vi "ROS2.vi"(7 "JPG":refnum<vi>, 10 "queueName":string="PV_script", 11 "Console Reference":refnum<vi>) -> ()   [LabVIEW 2022 SP3]
uses:
  ROS_Subs/ROSCtrl.ctl
  <vilib>/Platform/browser.llb/Open URL in Default Browser (string).vi
panel:
  in  "Tab Control":T1(tab)
  in  "Cmds":T2
  in  "LightShow":u32[](array[colorbox])=[16711680, 327424, 393471, 15699456, 14811391, 64255]
  in  "LED Colors":u32[](array[colorbox])=[16711680, 327424, 393471, 15699456, 14811391, 64255]
  in  "LED Info":T3={"Node Name"="Node", "Topic Name"="/cmd_lightring", "Message Type"="irobot_create_msgs/msg/LightringLeds", "Message"="{\"override_system\":true,\"leds\":[{\"red\":255,\"green\":0,\"blue\":0},{\"red\":4,\"green\":255,\"blue\":0},{\"red\":6,\"green\":0,\"blue\":255},{\"red\":239,\"green\":142,\"blue\":0},{\"red\":226,\"green\":0,\"blue\":255},{\"red\":0,\"green\":250,\"blue\":255}]}", "Pub_Time"="5"}
  in  "Battery Info":T3={"Node Name"="Node", "Topic Name"="/battery_state", "Message Type"="sensor_msgs/msg/BatteryState", "Message"="", "Pub_Time"="-1"}
  in  "Listener":T3={"Node Name"="Node", "Topic Name"="/chatter", "Message Type"="std_msgs/msg/String", "Message"="", "Pub_Time"="-1"}
  in  "Talker":T3={"Node Name"="Node", "Topic Name"="/chatter", "Message Type"="std_msgs/msg/String", "Message"="data:  Hi", "Pub_Time"="1"}
  in  "Try yourself":T4={"Node Name"="Node", "Topic Name"="/battery_state", "Message Type"="sensor_msgs/msg/BatteryState", "Message"="", "Pub_Time"="-1"}
  in  "Cmd Line":string
  out "Value":string
  in  "start":bool=TRUE
  in  "Send":bool
  out "Boolean":bool
  in  "Python":string="import rclpy\nfrom rclpy.node import Node\n\nfrom irobot_create_msgs.msg import LedColor\nimport irobot_create_msgs\n\nclass myPublisher(Node):\n    ''' Publish a custom color to each LED on the Create3 '''\n\n    def __init__(self, namespace: str = \"\"):\n        super().__init__('Node')\n        self.publisher = self.create_publisher(irobot_create_msgs.msg.LightringLeds, namespace + '/cmd_lightring', 10)\n\n        timer_period = 5 # seconds\n        self.timer = self.create_timer(timer_period, self.timer_callback)\n        self.payload = irobot_create_msgs.msg.LightringLeds()\n\n    def timer_callback(self):\n        '''This function will be called every 5 seconds '''\n        current_time = self.get_clock().now()\n\n        c0 = LedColor(red=255, green=0, blue=0)\n        c1 = LedColor(red=4, green=255, blue=0)\n        c2 = LedColor(red=6, green=0, blue=255)\n        c3 = LedColor(red=239, green=142, blue=0)\n        c4 = LedColor(red=226, green=0, blue=255)\n        c5 = LedColor(red=0, green=250, blue=255)\n        self.payload.override_system = True\n        self.payload.leds = [c0,c1,c2,c3,c4,c5]\n\n        self.payload.header.stamp = current_time.to_msg()\n        self.publisher.publish(self.payload)\n\ndef main():\n    rclpy.init()\n    publisher = myPublisher()\n\n    try:\n        rclpy.spin(publisher)\n    except KeyboardInterrupt:\n        print('\\nCaught Keyboard Interrupt')\n    finally:\n        print(\"Done\")\n        publisher.reset()\n        publisher.destroy_node()\n        rclpy.shutdown()\n\nmain()"
  # "Wrestling with ROS2"
  # "Publisher"
  # "-1 means \nsubscribe"
  # "Subscriber"
  # "-1 means \nsubscribe"
  # "/chatter"
  # "-1 means \nsubscribe"
  # "-1 means \nsubscribe"
  # "Try it yourself"
  # "-1 means \nsubscribe"
  # "ROS 2 Tutorials"
  # "https://docs.ros.org/en/galactic/Tutorials.html"
  # "https://github.com/paccionesawyer/Create3_Python/blob/7bb07a24225d0194804e37c53a89b5a2d3932fee/ROS2_Workshop/00_Create3_ROS2_Introduction.ipynb"
  # "Sawyer's Notebook"
  # "https://github.com/ubuntu-robotics/ros2_cheats_sheet/blob/master/cli/cli_cheats_sheet.pdf"
  # "A useful cheatsheet"
  # "rclpy API"
  # "https://docs.ros2.org/latest/api/rclpy/api.html"
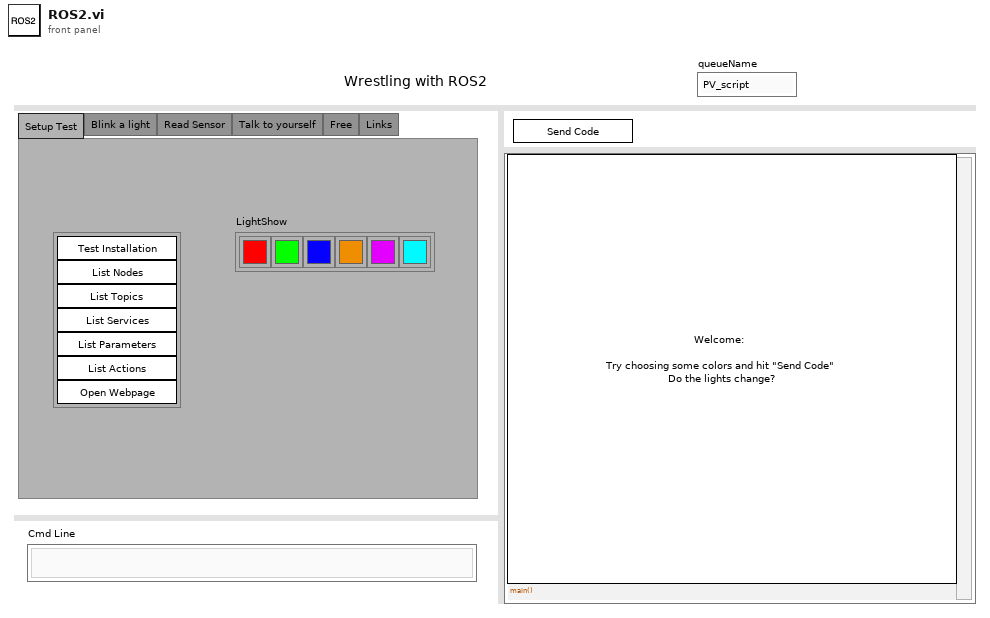
[diagram p1: front panel]
types:
  T1 = enum32{"Setup Test", "Blink a light", "Read Sensor", "Talk to yourself", "Free", "Links"}
  T2 = cluster{"doctor":bool, "Nodes":bool, "topics":bool, "services":bool, "params":bool, "actions":bool, "doctor 2":bool}
  T3 = typedef "ROSCtrl.ctl" = cluster{"Node Name":string, "Topic Name":string, "Message Type":string, "Message":string, "Pub_Time":string}
  T4 = cluster{"Node Name":string, "Topic Name":string, "Message Type":string, "Message":string, "Pub_Time":string}
  T5 = enum32{"Setup Test", "Blink a light", "Read Sensor", "Talk to yourself"}
  T6 = enum16{"read", "write pause", "write port", "write path", "write all"}
  T7 = cluster{"override_system":bool, "leds":cluster{"red":u8, "green":u8, "blue":u8}[]}
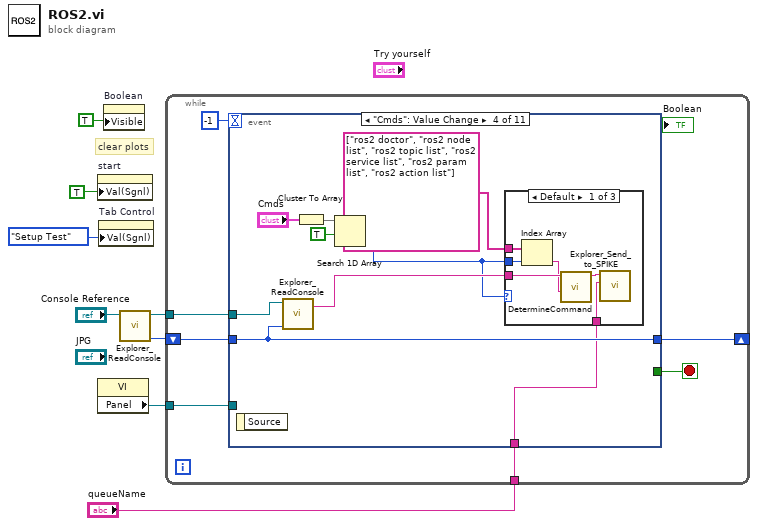
[diagram p0: block diagram]
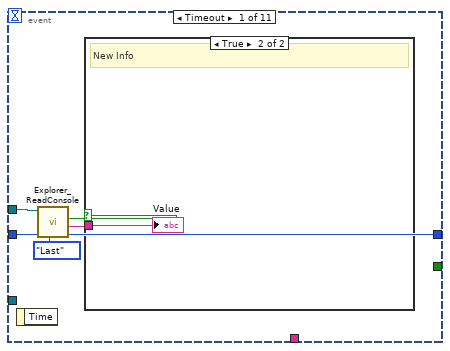
[diagram p2: hidden frame]
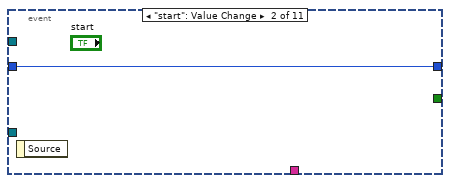
[diagram p4: hidden frame]
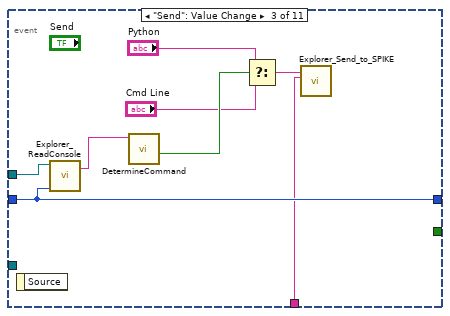
[diagram p5: hidden frame]
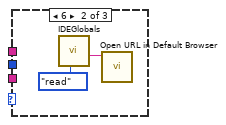
[diagram p6: hidden frame]
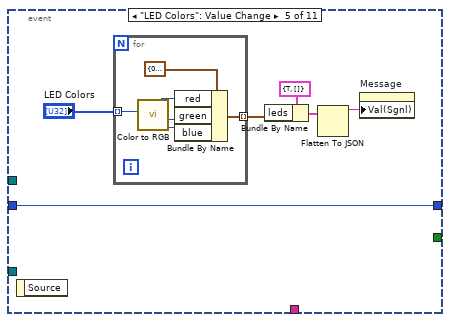
[diagram p8: hidden frame]
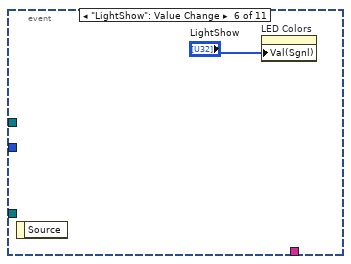
[diagram p9: hidden frame]
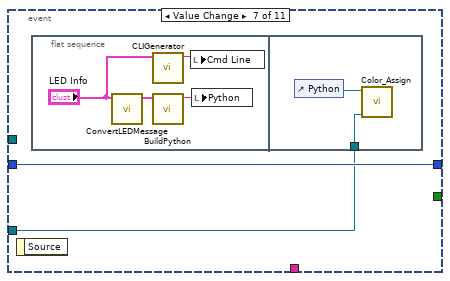
[diagram p10: hidden frame]
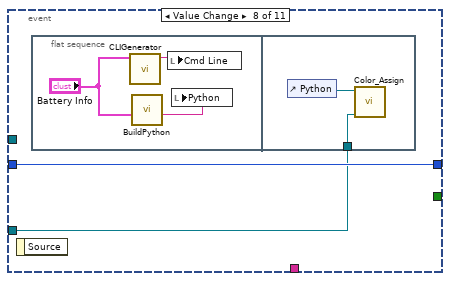
[diagram p11: hidden frame]
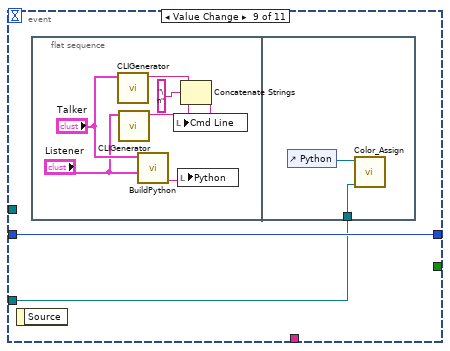
[diagram p12: hidden frame]
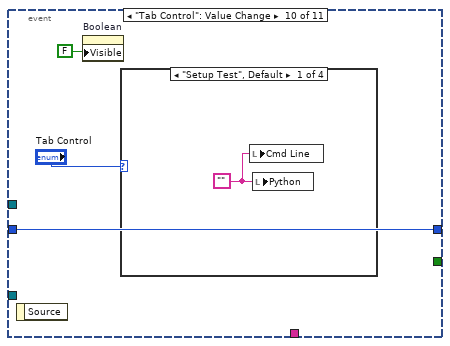
[diagram p13: hidden frame]
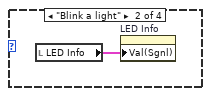
[diagram p14: hidden frame]
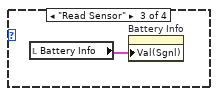
[diagram p15: hidden frame]
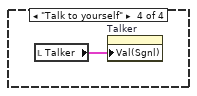
[diagram p16: hidden frame]
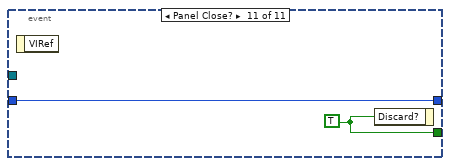
[diagram p17: hidden frame]
diagram:
  # "clear plots"
  n1 = property on="start" class="Bool (strict)"("Val(Sgnl)"=TRUE ("Value (Signaling)")) -> ()  [unwired: 2 in, 2 out]
  n2 = property class="VI"() -> ("Panel"=w4:refnum<vi>)  [unwired: 2 in, 2 out]
  n3 = property on="Tab Control" class="TabCtl (strict)"("Val(Sgnl)"=T5."Setup Test" ("Value (Signaling)")) -> ()  [unwired: 2 in, 2 out]
  n4 = property on="Boolean" class="Bool (strict)"("Visible"=TRUE) -> ()  [unwired: 2 in, 2 out]
  n5 = call "Explorer_ReadConsole.vi"("String in"="Console Reference") -> ("index out"=w7:i32, "String out"=w6:refnum<vi>)  [unwired: 6 in, 3 out]
  n6 = while {
    shift-right: [w13] -> _
    shift-left: w7 -> [w12]
    tunnel: w6 -> [w11]
    tunnel: w4 -> [w10]
    tunnel: "queueName" -> [w9]
    stop <- w14 stop-if-true
    n7 = event shown="[3] \"Cmds\": Value Change" {
      selector: _ -> [_ _ _ _ _ _ _ _ _ _ _]
      dyn-events: _ -> [_ _ _ _ _ _ _ _ _ _ _]
      timeout: -1 -> [_ _ _ _ _ _ _ _ _ _ _]
      tunnel: [_ _ _ _ _ _ _ _ _ _ w96] -> w14
      tunnel: [w20 w23 w30 w40 w54 _ w63 w71 w78 w90 w95] -> w13
      tunnel: w12 -> [w21 w23 w30 w40 w54 _ w63 w71 w78 w90 w95]
      tunnel: w11 -> [w17 _ w29 w39 _ _ _ _ _ _ _]
      tunnel: w10 -> [_ _ _ _ _ _ w62 w70 w77 _ _]
      tunnel: w9 -> [_ _ w24 w32 _ _ _ _ _ _ _]
      event Timeout {
        n8 = event-data() -> ()  [unwired: 1 in, 1 out]
        n9 = call "Explorer_ReadConsole.vi"("Reading"=enum16{"Next", "Last"}."Last" ("type"), "index in"=w21, "String in"=w17) -> ("index out"=w20:i32, "New Line"=w19:string, "New point?"=w18:bool)  [unwired: 4 in, 2 out]
        n10 = case shown="True" w18 {
          tunnel: w19 -> [_ w22]
          frame False {
            # "nothing new"
          }
          frame True {
            # "New Info"
            "Value" <- w22
          }
        }
      }
      event "start": Value Change {
        n11 = event-data() -> ()  [unwired: 1 in, 1 out]
      }
      event "Send": Value Change {
        n12 = event-data() -> ()  [unwired: 1 in, 1 out]
        n13 = call "Explorer_ReadConsole.vi"("index in"=w30, "String in"=w29) -> ("Value"=w31:string)  [unwired: 5 in, 4 out]
        n14 = call "DetermineCommand.vi"("Console"=w31) -> ("python?"=w28:bool)  [unwired: 9 in, 1 out]
        n15 = Select(t="Python", s=w28, f="Cmd Line") -> (s? t:f=w25:string)
        n16 = call "Explorer_Send_to_SPIKE.vi"("queueName"=w24, "python"=w25) -> ()  [unwired: 9 in, 1 out]
      }
      event "Cmds": Value Change {
        n17 = event-data() -> ()  [unwired: 1 in, 1 out]
        n18 = call "Explorer_ReadConsole.vi"("index in"=w40, "String in"=w39) -> ("Value"=w38:string)  [unwired: 5 in, 4 out]
        n19 = Cluster To Array(cluster="Cmds") -> (array=w36:bool[])
        n20 = Search 1D Array(1D array=w36, element=TRUE) -> (index of element=w33:i32)  [unwired: 1 in]
        n21 = case shown="Default" w33 {
          tunnel: w38 -> [w46 _ _]
          tunnel: string[] ["ros2 doctor", "ros2 node list", "ros2 topic list", "ros2 service list", "ros2 param list", "ros2 action list"] -> [w44 _ _]
          tunnel: w33 -> [w43 _ _]
          tunnel: w32 -> [w41 _ _]
          frame Default {
            n22 = Index Array(array=w44, index=w43) -> (element=w42:string)
            n23 = call "DetermineCommand.vi"("cmd"=w42, "Console"=w46) -> ("cmd out"=w45:string)  [unwired: 8 in, 1 out]
            n24 = call "Explorer_Send_to_SPIKE.vi"("queueName"=w41, "python"=w45) -> ()  [unwired: 9 in, 1 out]
          }
          frame 6 {
            n25 = call "IDEGlobals.vi"("task"=T6."read") -> ("Port out"=w47:string)  [unwired: 8 in, 2 out]
            n26 = call-poly <vilib>:"Open URL in Default Browser.vi"("URL"=w47) -> ()  [unwired: 5 in, 2 out]
          }
          frame -1 {
          }
        }
      }
      event "LED Colors": Value Change {
        n27 = event-data() -> ()  [unwired: 1 in, 1 out]
        n28 = for {
          tunnel: "LED Colors" -> [w60] mode=indexing
          tunnel: [w55] -> w51 mode=indexing
          n29 = call <vilib>:"Color to RGB.vi"("Color"=w60) -> ("R"=w58:u8, "G"=w57:u8, "B"=w56:u8)  [unwired: 1 out]
          n30 = Bundle By Name(cluster=cluster{"red":u8, "green":u8, "blue":u8} {"red"=0, "green"=0, "blue"=0}, "red"=w58, "green"=w57, "blue"=w56) -> (w55:cluster{"red":u8, "green":u8, "blue":u8})
        }
        n31 = Bundle By Name(cluster=T7 {"override_system"=TRUE, "leds"=[]}, "leds"=w51) -> (w50:T7)
        n32 = Flatten To JSON(anything=w50) -> (JSON string=w49:string)  [unwired: 2 in, 1 out]
        n33 = property on="Message" class="Str"("Val(Sgnl)"=w49) -> ()  [unwired: 2 in, 2 out]
      }
      event "LightShow": Value Change {
        n34 = event-data() -> ()  [unwired: 1 in, 1 out]
        n35 = property on="LED Colors" class="Arr (strict)"("Val(Sgnl)"="LightShow") -> ()  [unwired: 2 in, 2 out]
      }
      event Value Change {
        n36 = event-data() -> ()  [unwired: 1 in, 1 out]
        n37 = flat-sequence {
          tunnel: w62 -> [w68]
          frame #0 {
            n38 = call "ConvertLEDMessage.vi"("ROS Info"="LED Info") -> ("ROS corrected"=w66:T3)  [unwired: 10 in]
            n39 = call "CLIGenerator.vi"("ROS Info"="LED Info") -> ("CLI"=w65:string)  [unwired: 10 in]
            n40 = call "BuildPython.vi"("Publisher"=w66) -> ("result Pub"=w67:string)  [unwired: 8 in, 2 out]
            n41 = local write "Cmd Line"(w65) -> ()
            n42 = local write "Python"(w67) -> ()
          }
          frame #1 {
            n43 = control-ref of="Python"() -> (w69:refnum<vi>)
            n44 = call "Color_Assign.vi"("Front Panel"=w68, "Code"=w69) -> ()  [unwired: 9 in, 1 out]
          }
        }
      }
      event Value Change {
        n45 = event-data() -> ()  [unwired: 1 in, 1 out]
        n46 = flat-sequence {
          tunnel: w70 -> [w75]
          frame #0 {
            n47 = call "CLIGenerator.vi"("ROS Info"="Battery Info") -> ("CLI"=w74:string)  [unwired: 10 in]
            n48 = call "BuildPython.vi"("Subscriber"="Battery Info") -> ("result Sub"=w72:string)  [unwired: 8 in, 2 out]
            n49 = local write "Cmd Line"(w74) -> ()
            n50 = local write "Python"(w72) -> ()
          }
          frame #1 {
            n51 = control-ref of="Python"() -> (w76:refnum<vi>)
            n52 = call "Color_Assign.vi"("Front Panel"=w75, "Code"=w76) -> ()  [unwired: 9 in, 1 out]
          }
        }
      }
      event Value Change {
        n53 = event-data() -> ()  [unwired: 1 in, 1 out]
        n54 = flat-sequence {
          tunnel: w77 -> [w86]
          frame #0 {
            n55 = call "CLIGenerator.vi"("ROS Info"="Talker") -> ("CLI"=w83:string)  [unwired: 10 in]
            n56 = call "CLIGenerator.vi"("ROS Info"="Listener") -> ("CLI"=w82:string)  [unwired: 10 in]
            n57 = call "BuildPython.vi"("Subscriber"="Listener", "Publisher"="Talker") -> ("result both"=w79:string)  [unwired: 7 in, 2 out]
            n58 = local write "Python"(w79) -> ()
            n59 = Concatenate Strings(w83, "\n" ("string"), w82) -> (w80:string)
            n60 = local write "Cmd Line"(w80) -> ()
          }
          frame #1 {
            n61 = control-ref of="Python"() -> (w87:refnum<vi>)
            n62 = call "Color_Assign.vi"("Front Panel"=w86, "Code"=w87) -> ()  [unwired: 9 in, 1 out]
          }
        }
      }
      event "Tab Control": Value Change {
        n63 = event-data() -> ()  [unwired: 1 in, 1 out]
        n64 = property on="Boolean" class="Bool (strict)"("Visible"=FALSE) -> ()  [unwired: 2 in, 2 out]
        n65 = case shown="\"Setup Test\", Default" "Tab Control" {
          frame "Setup Test", Default {
            w91 = ""
            n66 = local write "Cmd Line"(w91) -> ()
            n67 = local write "Python"(w91) -> ()
          }
          frame "Blink a light" {
            n68 = local read "LED Info"() -> (w92:T3)
            n69 = property on="LED Info" class="Clust (strict)"("Val(Sgnl)"=w92) -> ()  [unwired: 2 in, 2 out]
          }
          frame "Read Sensor" {
            n70 = local read "Battery Info"() -> (w93:T3)
            n71 = property on="Battery Info" class="Clust (strict)"("Val(Sgnl)"=w93) -> ()  [unwired: 2 in, 2 out]
          }
          frame "Talk to yourself" {
            n72 = local read "Talker"() -> (w94:T3)
            n73 = property on="Talker" class="Clust (strict)"("Val(Sgnl)"=w94) -> ()  [unwired: 2 in, 2 out]
          }
        }
      }
      event Panel Close? {
        w96 = TRUE ("Discard?")
        n74 = event-data() -> ()  [unwired: 1 in, 1 out]
        n75 = event-data("Discard?"=w96) -> ()  [unwired: 1 in, 1 out]
      }
    }
  }
